vi "New from WAMP message.vi"(8 "error in (no error)":errorcluster, 11 "WampMessage MsgPack":refnum<class "WampMessage MsgPack.lvclass">) -> (0 "error out":errorcluster, 2 "Error data (MsgPack)":T1, 3 "ErrorHandler MsgPack out":refnum<class "ErrorHandler MsgPack.lvclass">)   [LabVIEW 2020, in "wamplv.lvlib" / "ErrorHandler MsgPack.lvclass"]
uses:
  ErrorHandler MsgPack.lvclass
  ErrorHandler MsgPack.lvclass/ErrorHandler MsgPack.ctl
  SerialisedMessages/MsgPackMessage/WampMessage MsgPack.lvclass
  TypeDefs/WAMP Message Codes.ctl
  wamplv.lvlib
  MessagePack/MsgPackArray/MsgPackArray.lvclass
  MessagePack/MsgPackMap/MsgPackMap.lvclass
  TypeDefs/Error or abort detail (MsgPack).ctl
  TypeDefs/Error data (MsgPack).ctl
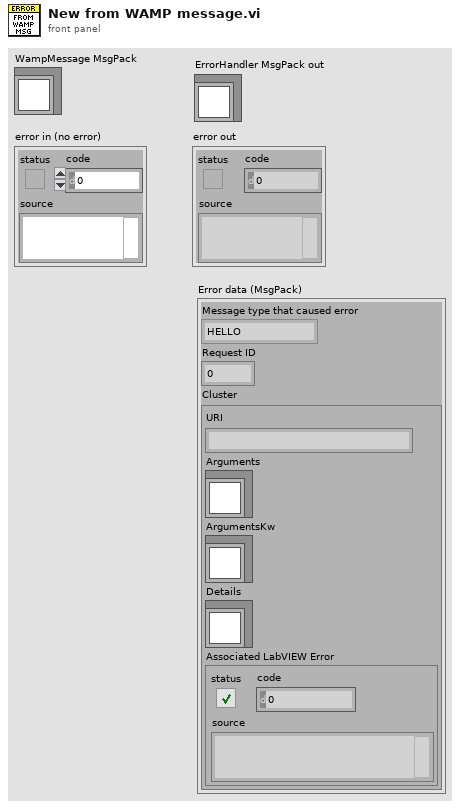
[diagram p1: front panel]
types:
  T1 = typedef "wamplv.lvlib/Error data (MsgPack).ctl" = cluster{"Message type that caused error":T2, "Request ID":u64, "Cluster":T3}
  T2 = typedef "wamplv.lvlib/WAMP Message Codes.ctl" = enum8{"HELLO", "WELCOME", "CHALLENGE", "AUTHENTICATE", "ABORT", "GOODBYE", "ERROR", "PUBLISH", "PUBLISHED", "SUBSCRIBE", "SUBSCRIBED", "UNSUBSCRIBE", "UNSUBSCRIBED", "EVENT", "CALL", "RESULT", "REGISTER", "REGISTERED", "UNREGISTER", "UNREGISTERED", "INVOCATION", "YIELD"}
  T3 = typedef "wamplv.lvlib/Error or abort detail (MsgPack).ctl" = cluster{"URI":string, "Arguments":refnum<class "MsgPackArray.lvclass">, "ArgumentsKw":refnum<class "MsgPackMap.lvclass">, "Details":refnum<class "MsgPackMap.lvclass">, "Associated LabVIEW Error":errorcluster}
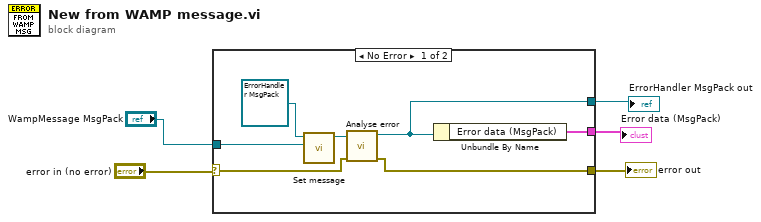
[diagram p0: block diagram]
diagram:
  n1 = case shown="No Error" "error in (no error)" {
    selector: "error in (no error)" -> [w8 w13]
    tunnel: [w7 _] -> w4
    tunnel: [w12 _] -> w1
    tunnel: "WampMessage MsgPack" -> [w10 _]
    tunnel: [w6 w13] -> w2
    frame No Error {
      n2 = call-dynamic "Set message.vi"("WampMessage MsgPack"=w10, "ErrorHandler MsgPack in"=refnum<class "ErrorHandler MsgPack.lvclass"> refnum ("wamplv.lvlib:ErrorHandler MsgPack.lvclass")) -> ("ErrorHandler MsgPack out"=w9:refnum<class "ErrorHandler MsgPack.lvclass">)  [unwired: 9 in]
      n3 = call-dynamic "Analyse error.vi"("error in (no error)"=w8, "IErrorHandler in"=w9) -> ("error out"=w6:errorcluster, "IErrorHandler out"=w7:refnum<class "ErrorHandler MsgPack.lvclass">)  [unwired: 8 in]
      n4 = Unbundle By Name(w7) -> ("Error data (MsgPack)"=w12:T1)
    }
    frame Error {
    }
  }
  "error out" <- w2
  "ErrorHandler MsgPack out" <- w4
  "Error data (MsgPack)" <- w1
